vi "Setup.vi"(5 "Protocol selection\n(appended)":T1 {"Mode" items=["Modbus-1", "3"]}, 7 "protocol selection ref":refnum<vi>, 8 "error in (no error)":errorcluster, 9 "search":bool, 10 "Comm master cluster in":T4={"Main event var"=refnum, "VIRef"=refnum, "Data path"=path "", "Reads"=0, "total number of UUT"=0, "FF refnum"={"Handle1"=0, "Handle2"=0}, "FF device id list"=[], "MODBUS resource name"="", "MODBUS Serial Parameters"={"Mode"=enum."RTU", "Default Slave Address"=0, "MODBUS timeout"=0, "Baud Rate"=0, "Parity"=0, "Flow Control"=0}, "Profibus resource name"="", "Profibus Communication ref.:"=0, "HART resource name"="", "HART long addresses (array)"=[], "Comm relay session"="", "Comm UI event"=refnum, "Write Interval (s)"=5.0, "DMM_QUEUE"=refnum, "POWER_QUEUE"=refnum, "\nTHERM_QUEUE"=refnum, "\nCOMM_QUEUE"=refnum, "TIMING_QUEUE"=refnum, "MAIN_QUEUE"=refnum, "Log path"=path ""} {"Write Interval (s)" min=0.1 max=1000.0 step=0.1}, 11 "MODBUS in":refnum<class "USB_MODBUS.lvclass">) -> (0 "error out":errorcluster, 3 "MODBUS out":refnum<class "USB_MODBUS.lvclass">)   [LabVIEW 2016, in "USB_MODBUS.lvclass"]
uses:
  USB_MODBUS.lvclass
  MASTER_OPC.ctl
  Typedef/event var.ctl
  Typedef/Comm ui action type.ctl
  Typedef/Comm_State_enum.ctl
  Typedef/state var.ctl
  Typedef/Array_of_Comm_mode_and_address_types.ctl
  Typedef/Comm_mode_and_address_type.ctl
  Typedef/Comm_mode_type_combo.ctl
  Typedef/Protocol_enum_type.ctl
  USB_MODBUS.lvclass/USB_MODBUS.ctl
  Protocol Class/Protocol.lvclass
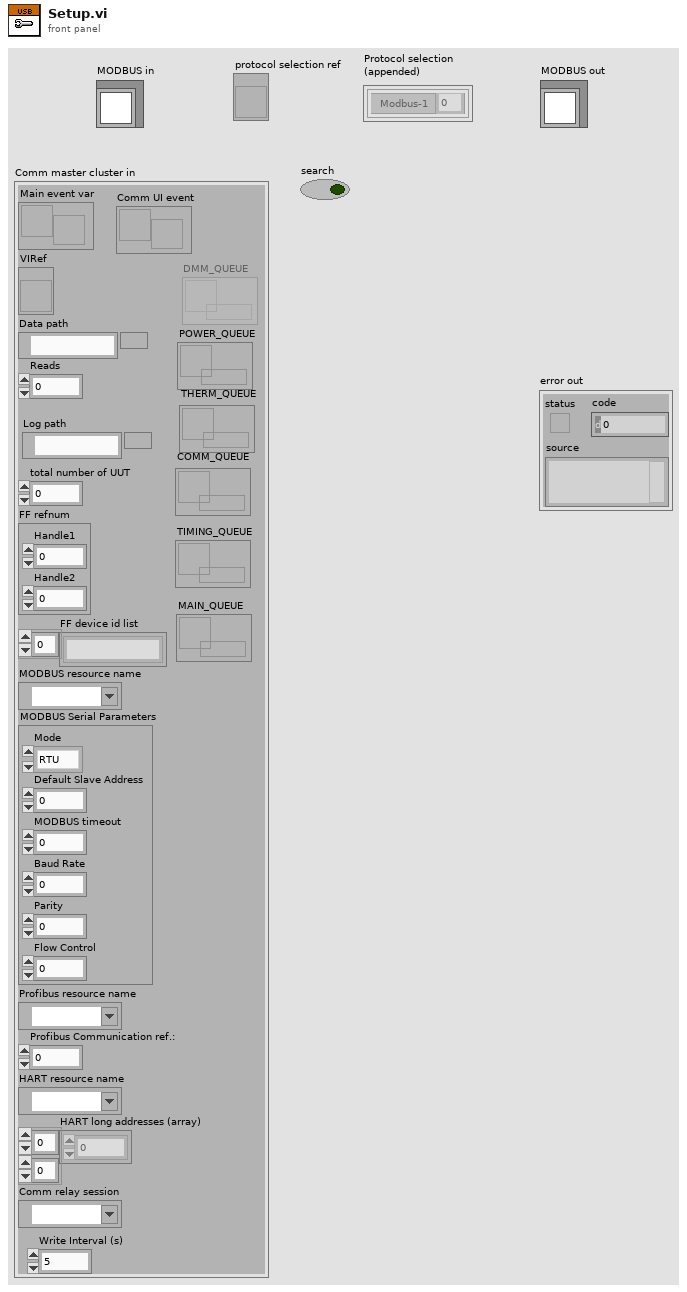
[diagram p1: front panel]
types:
  T1 = typedef "Array_of_Comm_mode_and_address_types.ctl" = T2[]
  T2 = typedef "Comm_mode_and_address_type.ctl" = cluster{"address":i32, "Mode":T3}
  T3 = typedef "Comm_mode_type_combo.ctl" = u16
  T4 = typedef "MASTER_OPC.ctl" = cluster{"Main event var":refnum<user-event>, "VIRef":refnum<vi>, "Data path":path, "Reads":i32, "total number of UUT":i32, "FF refnum":cluster{"Handle1":u32, "Handle2":u32}, "FF device id list":string[], "MODBUS resource name":refnum<visa-resource-name>, "MODBUS Serial Parameters":cluster{"Mode":enum16{"RTU", "ASCII"}, "Default Slave Address":u8, "MODBUS timeout":u32, "Baud Rate":u32, "Parity":u16, "Flow Control":u16}, "Profibus resource name":refnum<visa-resource-name>, "Profibus Communication ref.:":u8, "HART resource name":refnum<visa-resource-name>, "HART long addresses (array)":u8[][], "Comm relay session":refnum<k15>, "Comm UI event":refnum<user-event>, "Write Interval (s)":dbl, "DMM_QUEUE":refnum<queue>, "POWER_QUEUE":refnum<queue>, "\nTHERM_QUEUE":refnum<queue>, "\nCOMM_QUEUE":refnum<queue>, "TIMING_QUEUE":refnum<queue>, "MAIN_QUEUE":refnum<queue>, "Log path":path}
  T5 = typedef "Protocol_enum_type.ctl" = enum16{"None", "MODBUS", "HART", "Fieldbus", "Profibus DP", "Profibus PA", "DeviceNET", "USB"}
  T6 = enum16{"Connect whole bus", "Connect individual UUTs", "Connect none"}
  T7 = cluster{"Device address":i32, "Switch index":i32}
  T8 = typedef "MODBUS parameters type.ctl" = cluster{"Mode":enum16{"RTU", "ASCII"}, "Default Slave Address":u8, "MODBUS timeout":u32, "Baud Rate":u32, "Parity":u16, "Flow Control":u16}
  T9 = cluster{"Device address":i32, "Switch index":i32}[]
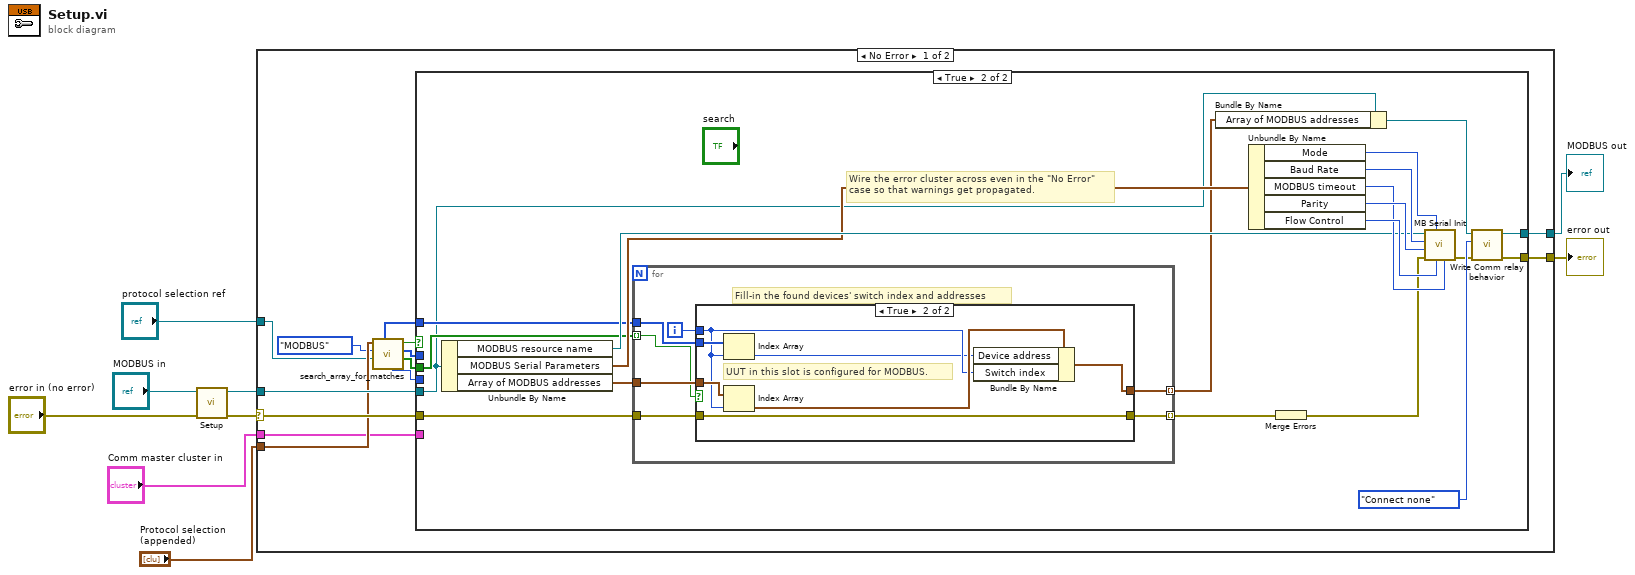
[diagram p0: block diagram]
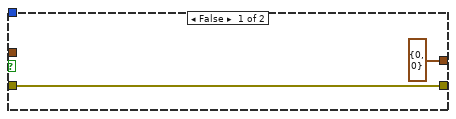
[diagram p3: hidden frame]
diagram:
  n1 = call-parent "Setup.vi"("error in (no error)"="error in (no error)", "Protocol in"="MODBUS in") -> ("error out"=w7:errorcluster, "Protocol out"=w5:refnum<class "USB_MODBUS.lvclass">)  [unwired: 8 in]
  n2 = case shown="No Error" w7 {
    selector: w7 -> [w22 w61]
    tunnel: [w21 w61] -> w6
    tunnel: w5 -> [w20 w62]
    tunnel: [w10 w62] -> w4
    tunnel: "Comm master cluster in" -> [w13 _]
    tunnel: "Protocol selection\n(appended)" -> [w19 _]
    tunnel: "protocol selection ref" -> [w18 _]
    frame No Error {
      n3 = call "search_array_for_matches.vi"("protocol selection ref"=w18, "Protocol enum"=Protocol_enum_type."MODBUS", "appended array"=w19) -> ("Array of exists"=w15:bool[], "array of indexes"=w11:i32[], "exists?"=w16:bool, "Switch Row"=w12:i32, "all addresses"=w14:i32[])  [unwired: 3 in, 1 out]
      n4 = case shown="True" w16 {
        tunnel: w22 -> [w24 w25]
        tunnel: [w24 w26] -> w21
        tunnel: w20 -> [w23 w31]
        tunnel: w14 -> [_ w34]
        tunnel: w15 -> [_ w35]
        tunnel: w13 -> [_ _]
        tunnel: w12 -> [_ _]
        tunnel: w11 -> [_ _]
        tunnel: [w23 w28] -> w10
        frame False {
        }
        frame True {
          # "Wire the error cluster across even in the \"No Error\"\ncase so that warnings get propagated."
          n5 = Unbundle By Name(w31) -> ("MODBUS resource name"=w39:refnum<visa-resource-name>, "MODBUS Serial Parameters"=w38:T8, "Array of MODBUS addresses"=w37:T9)
          n6 = for {
            tunnel: w37 -> [w51]
            tunnel: [w50] -> w32 mode=indexing
            tunnel: w25 -> [w49]
            tunnel: [w48] -> w36 mode=indexing
            tunnel: w35 -> [w47] mode=indexing
            tunnel: w34 -> [w45]
            i -> [w46]
            # "Fill-in the found devices' switch index and addresses"
            n7 = case shown="True" w47 {
              tunnel: w51 -> [_ w60]
              tunnel: w45 -> [_ w59]
              tunnel: [T7 {"Device address"=0, "Switch index"=0} ("Hart address") w54] -> w50
              tunnel: w49 -> [w53 w56]
              tunnel: [w53 w56] -> w48
              tunnel: w46 -> [_ w57]
              frame False {
              }
              frame True {
                # "UUT in this slot is configured for MODBUS."
                n8 = Index Array(array=w59, index=w57) -> (element=w55:i32)
                n9 = Index Array(array=w60, index=w57) -> (element=w58:T7)
                n10 = Bundle By Name(cluster=w58, "Device address"=w55, "Switch index"=w57) -> (w54:T7)
              }
            }
          }
          n11 = Bundle By Name(cluster=w31, "Array of MODBUS addresses"=w32) -> (w30:refnum<class "USB_MODBUS.lvclass">)
          n12 = Unbundle By Name(w38) -> ("Mode"=w44:enum16{"RTU", "ASCII"}, "Baud Rate"=w43:u32, "MODBUS timeout"=w40:u32, "Parity"=w42:u16, "Flow Control"=w41:u16)
          n13 = Merge Errors(w36) -> (w33:errorcluster)
          n14 = call "MB Serial Init.vi"("Timeout"=w40, "Flow Control"=w41, "Mode"=w44, "error in (no error)"=w33, "Parity"=w42, "Baud Rate"=w43, "VISA resource name"=w39) -> ("error out"=w27:errorcluster)  [unwired: 4 out]
          n15 = call-dynamic "Write Comm relay behavior.vi"("error in (no error)"=w27, "Comm relay behavior"=T6."Connect none", "Protocol in"=w30) -> ("error out"=w26:errorcluster, "Protocol out"=w28:refnum<class "USB_MODBUS.lvclass">)  [unwired: 7 in]
        }
      }
    }
    frame Error {
    }
  }
  "error out" <- w6
  "MODBUS out" <- w4
